vi "DbaseCreateInitalFiles_BIN.vi"(8 "error in (no error)":errorcluster, 9 "DB_SetupData":T2 {"initial TAGs information"."Range L" format="%#_6p"; "initial TAGs information"."Range H" format="%#_6p"}, 11 "FAMM in":T3={"FAMM_PAQ_Layers"=0, "FAMM_PAQ_resolution"=0.0, "PAQ_TAGs"=[], "WAQ_TAGs"=[], "EAQ_TAGs"=[], "All_TAGs"=[], "PAQtagProps"=[], "WAQtagProps"=[], "EAQtagProps"=[], "DBAL_class"=refnum, "PAQ_memory"=[], "PAQupdates"=[], "FAMM_Size"={"other"=0, "1day"=0, "1week"=0}, "DatabaseFileExtention"="", "DatabaseSaveRate"=0.0, "Database_path"=path "G:/Sgraph_database", "DBAL-Queue"=refnum, "OS_name"="undefined"} {"FAMM_Size"."1week" format="%.0p"; "FAMM_Size"."1day" format="%.0p"; "FAMM_Size"."other" format="%.0p"; "EAQtagProps"."TagFunc" format="%08x"; "EAQtagProps"."RangeL" format="%.2f"; "EAQtagProps"."RangeH" format="%.2f"; "WAQtagProps"."TagFunc" format="%08x"; "WAQtagProps"."RangeL" format="%.2f"; "WAQtagProps"."RangeH" format="%.2f"; "PAQtagProps"."TagFunc" format="%08x"; "PAQtagProps"."RangeL" format="%.2f"; "PAQtagProps"."RangeH" format="%.2f"; "FAMM_PAQ_resolution" format="%.1p"}) -> (0 "error out":errorcluster, 3 "FAMM out":T3={"FAMM_PAQ_Layers"=0, "FAMM_PAQ_resolution"=0.0, "PAQ_TAGs"=[], "WAQ_TAGs"=[], "EAQ_TAGs"=[], "All_TAGs"=[], "PAQtagProps"=[], "WAQtagProps"=[], "EAQtagProps"=[], "DBAL_class"=refnum, "PAQ_memory"=[], "PAQupdates"=[], "FAMM_Size"={"other"=0, "1day"=0, "1week"=0}, "DatabaseFileExtention"="", "DatabaseSaveRate"=0.0, "Database_path"=path "G:/Sgraph_database", "DBAL-Queue"=refnum, "OS_name"="undefined"} {"FAMM_Size"."1week" format="%.0p"; "FAMM_Size"."1day" format="%.0p"; "FAMM_Size"."other" format="%.0p"; "EAQtagProps"."TagFunc" format="%08x"; "EAQtagProps"."RangeL" format="%.2f"; "EAQtagProps"."RangeH" format="%.2f"; "WAQtagProps"."TagFunc" format="%08x"; "WAQtagProps"."RangeL" format="%.2f"; "WAQtagProps"."RangeH" format="%.2f"; "PAQtagProps"."TagFunc" format="%08x"; "PAQtagProps"."RangeL" format="%.2f"; "PAQtagProps"."RangeH" format="%.2f"; "FAMM_PAQ_resolution" format="%.1p"})   [LabVIEW 2020, in "Sgraph_lib_V1.lvlib" / "FAMM.lvclass"]
doc: "Check if the database exists,\nIf yes and content is OK: then continue.\n\nIf parts are missing: Start user dialog and request what to do."
uses:
  FAMM.lvclass
  controls/FAMM-attributes.ctl
  Common/controls/typedef_com_TagProp.ctl
  DBAL/DBAL.lvclass
  PAQ-memory.lvclass
  DBAL/controls/DBAL_Command.ctl
  DBAL/controls/DBAL-commands.ctl
  controls/FAMM_DB_New_BIN_taginfo.ctl
  DBAL/controls/DBAL_TAGpropEdit.ctl
  Gview/controls/Typedef-PresetFileFormat.ctl
  Gview/controls/EditTagOneTag.ctl
  Gview/methods/GV_Typedef_PresetSaveSettings.ctl
  Gview/controls/Typedef_Live.ctl
  Gview/controls/Typedef_Autoscale.ctl
  Gview/controls/LegendSet.ctl
  <vilib>/Utility/miscctls.llb/LVPositionTypeDef.ctl
  <vilib>/Utility/miscctls.llb/LVBoundsTypeDef.ctl
  Gview/controls/YgraphDef.ctl
  Gview/controls/AutoScale.ctl
  Gview/controls/MinMax.ctl
  Gview/controls/TD_Lscale.ctl
  Gview/controls/TD_Rscale.ctl
  Builds/Sgraph_lib_V1.lvlib
  Gview/Gviewer.lvclass
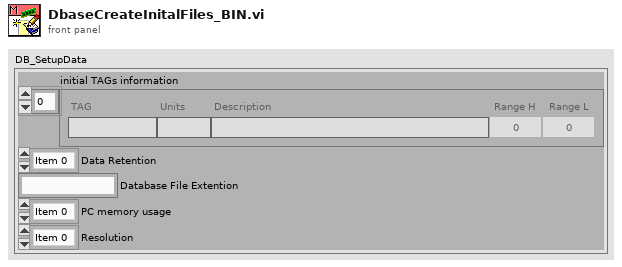
[diagram p1: front panel]
types:
  T1 = typedef "Sgraph_lib_V1.lvlib/FAMM.lvclass/FAMM_DB_New_BIN_taginfo.ctl" = cluster{"TAG":string, "Units":string, "Description":string, "Range H":dbl, "Range L":dbl}
  T2 = cluster{"initial TAGs information":T1[], "Data Retention":enum32{"Item 0", "Item 1", "Item 2", "Item 3", "Item 4"}, "Database File Extention":string, "PC memory usage":enum32{"Item 0", "Item 1", "Item 2", "Item 3", "Item 4"}, "Resolution":enum32{"Item 0", "Item 1", "Item 2", "Item 3", "Item 4"}}
  T3 = typedef "Sgraph_lib_V1.lvlib/FAMM.lvclass/FAMM-attributes.ctl" = cluster{"FAMM_PAQ_Layers":i32, "FAMM_PAQ_resolution":dbl, "PAQ_TAGs":string[], "WAQ_TAGs":string[], "EAQ_TAGs":string[], "All_TAGs":string[], "PAQtagProps":T4[], "WAQtagProps":T4[], "EAQtagProps":T4[], "DBAL_class":refnum<data-value>, "PAQ_memory":refnum<data-value>[], "PAQupdates":timestamp[], "FAMM_Size":cluster{"other":i32, "1day":i32, "1week":i32}, "DatabaseFileExtention":string, "DatabaseSaveRate":dbl, "Database_path":path, "DBAL-Queue":refnum<queue>, "OS_name":string}
  T4 = typedef "Sgraph_lib_V1.lvlib/typedef_com_TagProp.ctl" = cluster{"Description":string, "EngUnits":string, "RangeH":dbl, "RangeL":dbl, "Resolution":i32, "Obsolete":bool, "ChangeDate":timestamp, "ChangeSource":string, "ChangeReason":string, "TagFunc":u32}
  T5 = typedef "Sgraph_lib_V1.lvlib/DBAL.lvclass/DBAL_TAGpropEdit.ctl" = cluster{"TAG":string, "Qtype":string, "TAGprop":T4}
  T6 = typedef "Sgraph_lib_V1.lvlib/Gviewer.lvclass/EditTagOneTag.ctl" = cluster{"TAG":string, "min":dbl, "max":dbl, "Color":u32}
  T7 = cluster{"Save time?":bool, "Presets":T6[], "PresetFilePath":path}
  T8 = enum16{"big-endian, network order", "native, host order", "little-endian"}
  T9 = typedef "Sgraph_lib_V1.lvlib/Gviewer.lvclass/Typedef-PresetFileFormat.ctl" = cluster{"Time-Start":timestamp, "Time-End":timestamp, "Time-File":timestamp, "PresetSave":cluster{"Save time?":bool, "Presets":T6[], "PresetFilePath":path}, "PresetSaveSettings":T10}
  T10 = typedef "Sgraph_lib_V1.lvlib/Gviewer.lvclass/GV_Typedef_PresetSaveSettings.ctl" = cluster{"Live":T11, "Autoscale":T12, "Legend":T13, "Yscales":T16[], "YscaleMatch":bool, "AutoScale":T17, "AutoscaleContinuous":bool, "YscaleUseMinMax":bool, "MinMax":T18, "Lscale":T19, "Rscale":T20}
  T11 = typedef "Sgraph_lib_V1.lvlib/Gviewer.lvclass/Typedef_Live.ctl" = enum16{"Live View", "Freeze"}
  T12 = typedef "Sgraph_lib_V1.lvlib/Gviewer.lvclass/Typedef_Autoscale.ctl" = enum16{"Off", "Max", "Stack", "Norm"}
  T13 = typedef "Sgraph_lib_V1.lvlib/Gviewer.lvclass/LegendSet.ctl" = cluster{"Position":T14, "Size":T15, "Rows":u32, "Select":i32, "Visible":bool}
  T14 = typedef "LVPositionTypeDef.ctl" = cluster{"Left":i32, "Top":i32}
  T15 = typedef "LVBoundsTypeDef.ctl" = cluster{"Width":u32, "Height":u32}
  T16 = typedef "Sgraph_lib_V1.lvlib/Gviewer.lvclass/YgraphDef.ctl" = cluster{"Plot":i32, "X(%)":dbl}
  T17 = typedef "Sgraph_lib_V1.lvlib/Gviewer.lvclass/AutoScale.ctl" = enum16{"FitEqual", "FitMax", "StackEqual", "StackMax", "StackPerType"}
  T18 = typedef "Sgraph_lib_V1.lvlib/Gviewer.lvclass/MinMax.ctl" = enum16{"On", "Off", "Focus"}
  T19 = typedef "Sgraph_lib_V1.lvlib/Gviewer.lvclass/TD_Lscale.ctl" = enum16{"none", "one", "many"}
  T20 = typedef "Sgraph_lib_V1.lvlib/Gviewer.lvclass/TD_Rscale.ctl" = enum16{"none", "one", "all"}
  T21 = enum32{"Item 0", "Item 1", "Item 2", "Item 3", "Item 4"}
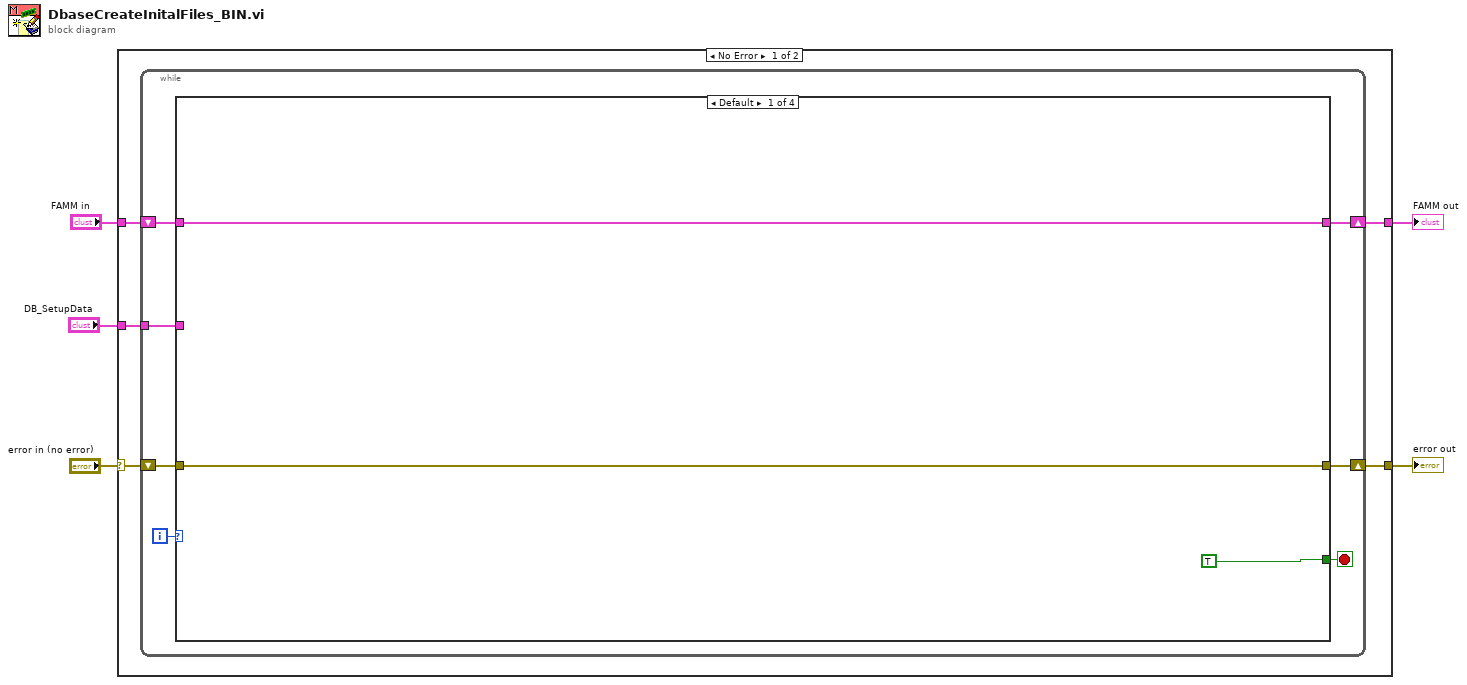
[diagram p0: block diagram]
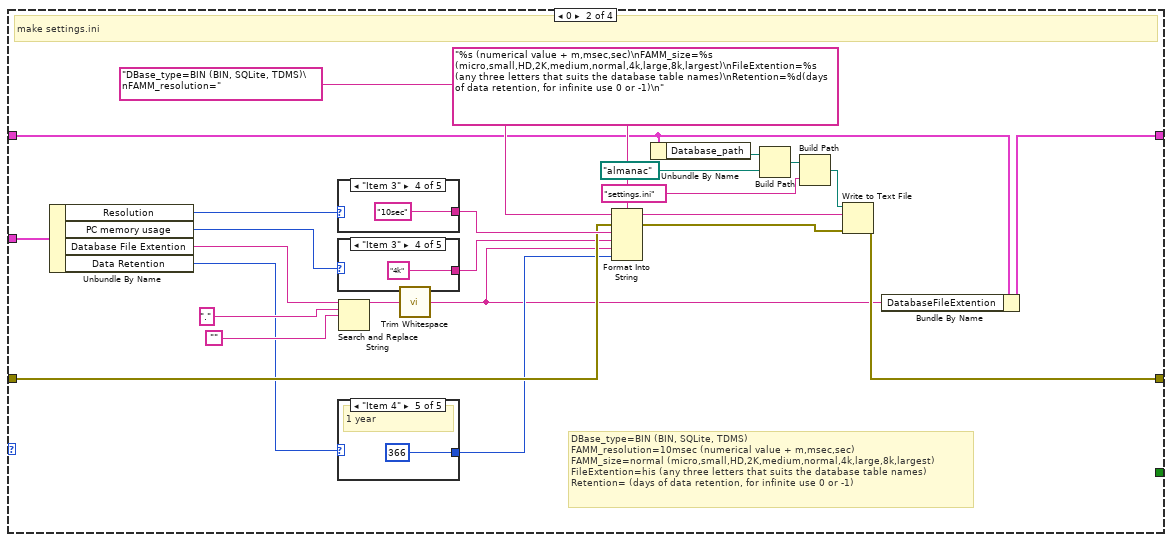
[diagram p2: hidden frame]
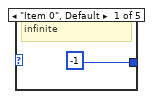
[diagram p3: hidden frame]
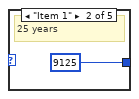
[diagram p4: hidden frame]
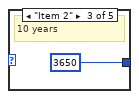
[diagram p5: hidden frame]
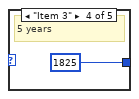
[diagram p6: hidden frame]
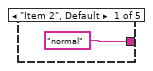
[diagram p7: hidden frame]
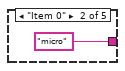
[diagram p8: hidden frame]
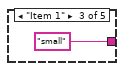
[diagram p9: hidden frame]
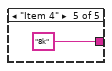
[diagram p10: hidden frame]
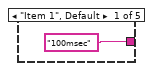
[diagram p11: hidden frame]
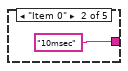
[diagram p12: hidden frame]
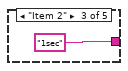
[diagram p13: hidden frame]
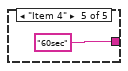
[diagram p14: hidden frame]
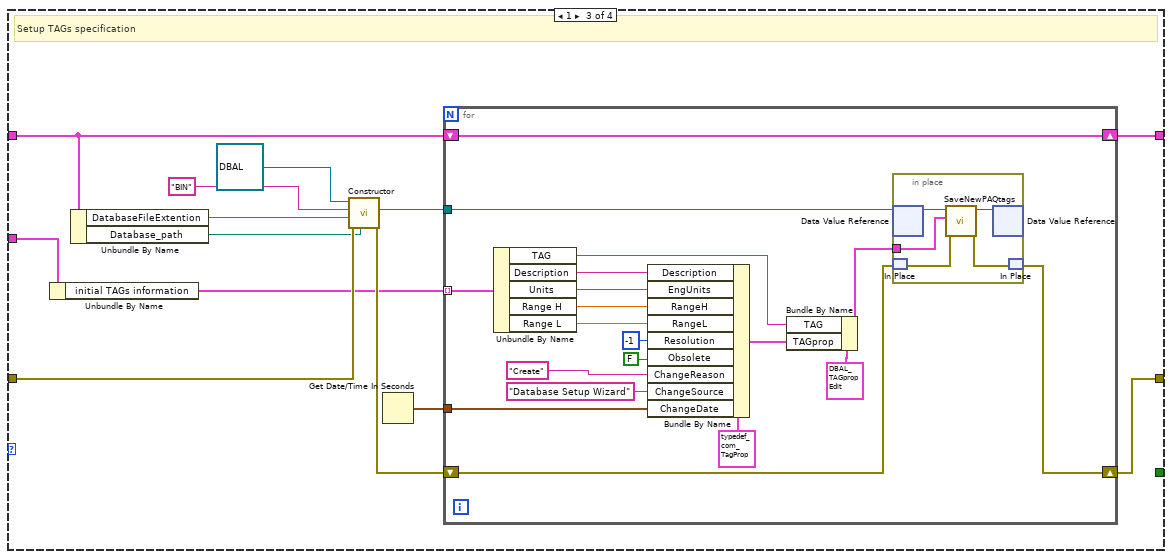
[diagram p15: hidden frame]
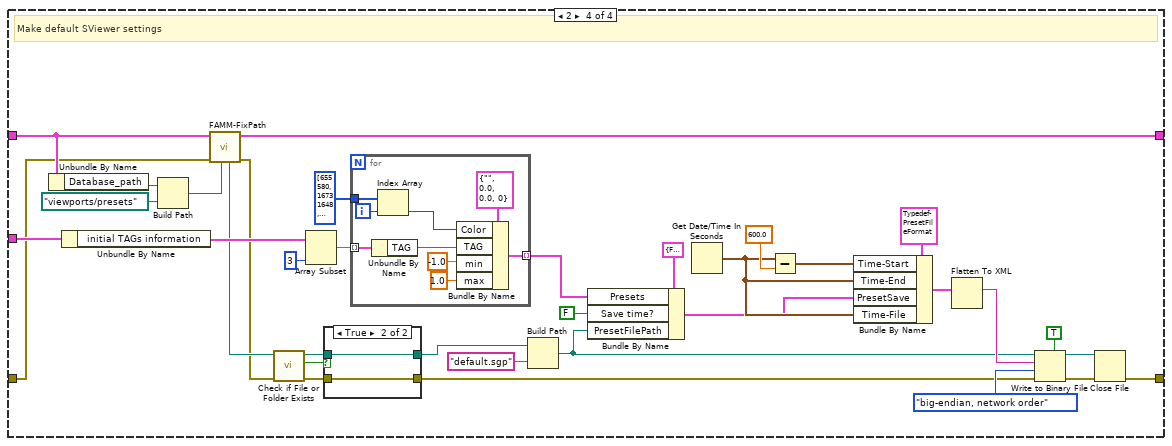
[diagram p16: hidden frame]
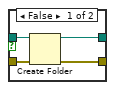
[diagram p17: hidden frame]
diagram:
  n1 = case shown="No Error" "error in (no error)" {
    selector: "error in (no error)" -> [w8 w149]
    tunnel: [w7 w149] -> w5
    tunnel: [w6 w148] -> w3
    tunnel: "FAMM in" -> [w9 w148]
    tunnel: "DB_SetupData" -> [w10 _]
    frame No Error {
      n2 = while {
        tunnel: w10 -> [w17]
        shift-right: [w14] -> w6
        shift-left: w9 -> [w15]
        shift-right: [w12] -> w7
        shift-left: w8 -> [w13]
        i -> [w16]
        stop <- w11 stop-if-true
        n3 = case shown="Default" w16 {
          tunnel: w17 -> [_ w45 w62 w114]
          tunnel: [w20 w22 w63 w103] -> w14
          tunnel: w15 -> [w20 w21 w64 w102]
          tunnel: w13 -> [w19 w40 w72 w98]
          tunnel: [w19 w24 w65 w125] -> w12
          tunnel: [TRUE _ _ _] -> w11
          frame Default {
          }
          frame 0 {
            # "DBase_type=BIN (BIN, SQLite, TDMS)\nFAMM_resolution=10msec (numerical value + m,msec,sec)\nFAMM_size=normal (micro,small,HD,2K,medium,normal,4k,large,8k,largest)\nFileExtention=his (any three letters that suits the database table names)\nRetention= (days of data retention, for infinite use 0 or -1)"
            # "make settings.ini"
            n4 = Unbundle By Name(w45) -> ("Resolution"=w43:T21, "PC memory usage"=w39:T21, "Database File Extention"=w37:string, "Data Retention"=w33:T21)
            n5 = case shown="\"Item 3\"" w43 {
              tunnel: ["100msec" "10msec" "1sec" "10sec" "60sec"] -> w42
              frame "Item 1", Default {
              }
              frame "Item 0" {
              }
              frame "Item 2" {
              }
              frame "Item 3" {
              }
              frame "Item 4" {
              }
            }
            n6 = case shown="\"Item 3\"" w39 {
              tunnel: ["normal" "micro" "small" "4k" "8k"] -> w38
              frame "Item 2", Default {
              }
              frame "Item 0" {
              }
              frame "Item 1" {
              }
              frame "Item 3" {
              }
              frame "Item 4" {
              }
            }
            n7 = case shown="\"Item 4\"" w33 {
              tunnel: [-1 9125 3650 1825 366] -> w32
              frame "Item 0", Default {
                # "infinite"
              }
              frame "Item 1" {
                # "25 years"
              }
              frame "Item 2" {
                # "10 years"
              }
              frame "Item 3" {
                # "5 years"
              }
              frame "Item 4" {
                # "1 year"
              }
            }
            n8 = Search and Replace String(input string=w37, search string=".", replace string="") -> (result string=w34:string)  [unwired: 5 in, 3 out]
            n9 = call <vilib>:"Trim Whitespace.vi"("string"=w34) -> ("trimmed string"=w23:string)  [unwired: 1 in]
            n10 = Format Into String(format string="%s (numerical value + m,msec,sec)\nFAMM_size=%s (micro,small,HD,2K,medium,normal,4k,large,8k,largest)\nFileExtention=%s (any three letters that suits the database table names)\nRetention=%d(days of data retention, for infinite use 0 or -1)\n" ("initial string"), initial string="DBase_type=BIN (BIN, SQLite, TDMS)\nFAMM_resolution=", error in=w40, w42, w38, w23, w32) -> (resulting string=w26:string, error out=w25:errorcluster)
            n11 = Unbundle By Name(w21) -> ("Database_path"=w31:path)
            n12 = Build Path(base path=w31, name or relative path=path "almanac") -> (appended path=w29:path)
            n13 = Build Path(base path=w29, name or relative path="settings.ini") -> (appended path=w27:path)
            n14 = Write to Text File(file (use dialog)=w27, text=w26, error in=w25) -> (error out=w24:errorcluster)  [unwired: 1 in, 2 out]
            n15 = Bundle By Name(cluster=w21, "DatabaseFileExtention"=w23) -> (w22:T3)
          }
          frame 1 {
            # "Setup TAGs specification"
            n16 = Unbundle By Name(w62) -> ("initial TAGs information"=w61:T1[])
            n17 = Unbundle By Name(w64) -> ("DatabaseFileExtention"=w71:string, "Database_path"=w69:path)
            n18 = call "Constructor.vi"("Database_location"=w69, "error in (no error)"=w72, "File extention"=w71, "DatabaseType"="BIN", "DBAL in"=refnum<class "DBAL.lvclass"> refnum) -> ("error out"=w66:errorcluster, "DBAL_class"=w67:refnum<data-value>)  [unwired: 4 in, 1 out]
            n19 = Get Date/Time In Seconds() -> (seconds since 1Jan1904=w68:timestamp)
            n20 = for {
              shift-right: [w84] -> w63
              shift-left: w64 -> [w84]
              shift-right: [w85] -> w65
              shift-left: w66 -> [w82]
              tunnel: w68 -> [w81]
              tunnel: w67 -> [w83]
              tunnel: w61 -> [w80] mode=indexing
              n21 = Unbundle By Name(w80) -> ("TAG"=w79:string, "Description"=w78:string, "Units"=w77:string, "Range H"=w76:dbl, "Range L"=w75:dbl)
              n22 = Bundle By Name(cluster=T4 {"Description"="", "EngUnits"="", "RangeH"=0.0, "RangeL"=0.0, "Resolution"=0, "Obsolete"=FALSE, "ChangeDate"=timestamp(0 s since 1904-01-01), "ChangeSource"="", "ChangeReason"="", "TagFunc"=0} ("TAGprop"), "Description"=w78, "EngUnits"=w77, "RangeH"=w76, "RangeL"=w75, "Resolution"=-1, "Obsolete"=FALSE, "ChangeReason"="Create", "ChangeSource"="Database Setup Wizard", "ChangeDate"=w81) -> (w87:T4)
              n23 = Bundle By Name(cluster=T5 {"TAG"="", "Qtype"="", "TAGprop"={"Description"="", "EngUnits"="", "RangeH"=0.0, "RangeL"=0.0, "Resolution"=0, "Obsolete"=FALSE, "ChangeDate"=timestamp(0 s since 1904-01-01), "ChangeSource"="", "ChangeReason"="", "TagFunc"=0}} ("TAGpropertyEdit"), "TAG"=w79, "TAGprop"=w87) -> (w86:T5)
              n24 = in-place {
                in-place-border: w86 -> [w93]
                n25 = in-place-dvr #1(w83) -> (w97:refnum<class "DBAL.lvclass">)  [unwired: 1 out]
                n26 = in-place-match #2(w82) -> (w96:errorcluster)
                n27 = call-dynamic "SaveNewPAQtags.vi"("error in (no error)"=w96, "TAGpropertyEdit"=w93, "DBAL in"=w97) -> ("error out"=w95:errorcluster, "DBAL out"=w94:refnum<class "DBAL.lvclass">)  [unwired: 7 in]
                n28 = in-place-dvr #1(w94) -> ()  [unwired: 2 out]
                n29 = in-place-match #2(w95) -> (w85:errorcluster)
              }
            }
          }
          frame 2 {
            # "Make default SViewer settings"
            n30 = Unbundle By Name(w102) -> ("Database_path"=w118:path)
            n31 = Unbundle By Name(w114) -> ("initial TAGs information"=w113:T1[])
            n32 = Build Path(base path=w118, name or relative path=path "viewports/presets") -> (appended path=w101:path)
            n33 = call "FAMM-FixPath.vi"("path-IN"=w101, "error in (no error)"=w98, "FAMM in"=w102) -> ("error out"=w99:errorcluster, "FAMM out"=w103:T3, "path-OUT"=w100:path)  [unwired: 6 in]
            n34 = call <vilib>:"Check if File or Folder Exists.vi"("error in (no error)"=w99, "path"=w100) -> ("error out"=w105:errorcluster, "file or folder exists?"=w108:bool, "dup path"=w107:path)  [unwired: 7 in]
            n35 = Array Subset(array=w113, length=3) -> (w111:T1[])  [unwired: 1 in]
            n36 = case shown="True" w108 {
              tunnel: w107 -> [w136 w138]
              tunnel: [w134 w138] -> w106
              tunnel: w105 -> [w135 w137]
              tunnel: [w133 w137] -> w104
              frame False {
                n37 = Create Folder(path (use dialog)=w136, error in=w135) -> (created path=w134:path, error out=w133:errorcluster)  [unwired: 1 in, 1 out]
              }
              frame True {
              }
            }
            n38 = for {
              tunnel: w111 -> [w147] mode=indexing
              tunnel: [w142] -> w110 mode=indexing
              tunnel: u32[] [655580, 16731648, 35073] -> [w141]
              i -> [w140]
              n39 = Unbundle By Name(w147) -> ("TAG"=w145:string)
              n40 = Index Array(array=w141, index=w140) -> (element=w139:u32)
              n41 = Bundle By Name(cluster=T6 {"TAG"="", "min"=0.0, "max"=0.0, "Color"=0} ("Selected-Tag"), "Color"=w139, "TAG"=w145, "min"=-1.0, "max"=1.0) -> (w142:T6)
            }
            n42 = Build Path(base path=w106, name or relative path="default.sgp") -> (appended path=w115:path)
            n43 = Bundle By Name(cluster=T7 {"Save time?"=FALSE, "Presets"=[], "PresetFilePath"=path ""} ("PresetSave"), "Presets"=w110, "Save time?"=FALSE, "PresetFilePath"=w115) -> (w120:T7)
            n44 = Get Date/Time In Seconds() -> (seconds since 1Jan1904=w122:timestamp)
            n45 = Subtract(x=w122, y=600.0) -> (x-y=w123:timestamp)
            n46 = Bundle By Name(cluster=T9 {"Time-Start"=timestamp(0 s since 1904-01-01), "Time-End"=timestamp(0 s since 1904-01-01), "Time-File"=timestamp(0 s since 1904-01-01), "PresetSave"={"Save time?"=FALSE, "Presets"=[], "PresetFilePath"=path ""}, "PresetSaveSettings"={"Live"=enum."Live View", "Autoscale"=enum."Off", "Legend"={"Position"={"Left"=0, "Top"=0}, "Size"={"Width"=0, "Height"=0}, "Rows"=0, "Select"=0, "Visible"=FALSE}, "Yscales"=[], "YscaleMatch"=FALSE, "AutoScale"=enum."FitEqual", "AutoscaleContinuous"=FALSE, "YscaleUseMinMax"=FALSE, "MinMax"=enum."On", "Lscale"=enum."none", "Rscale"=enum."none"}} ("PresetFileFormat"), "Time-Start"=w123, "Time-End"=w122, "PresetSave"=w120, "Time-File"=w122) -> (w131:T9)
            n47 = Flatten To XML(6:w131) -> (2:w129:string)
            n48 = Write to Binary File(file (use dialog)=w115, data=w129, error in=w104, 5:TRUE ("prepend array or string size? (T)"), 9:T8."big-endian, network order" ("byte order (0:big-endian, network order)")) -> (refnum out=w127:refnum<file>, error out=w126:errorcluster)  [unwired: 1 in, 1 out]
            n49 = Close File(refnum=w127, error in=w126) -> (error out=w125:errorcluster)  [unwired: 1 out]
          }
        }
      }
    }
    frame Error {
    }
  }
  "error out" <- w5
  "FAMM out" <- w3
